vi "Read Attributes.vi"(11 "Set DER GenerationMode Msg":refnum<class "Set DER GenerationMode Msg.lvclass">) -> (2 "Payload":cluster{"DER_setGenerationMode":T1})   [LabVIEW 2018, in "Device Communication and Control Abstract Actor.lvlib" / "Set DER GenerationMode Msg.lvclass"]
uses:
  Set DER GenerationMode Msg.lvclass
  <vilib>/ORNL/CSEISMIC DDS/CSEISMIC DDS Base/Data Types/DER_setGenerationMode.ctl
  <vilib>/ORNL/CSEISMIC DDS/CSEISMIC DDS Base/Data Types/Controls/DeviceID.ctl
  <vilib>/ORNL/CSEISMIC DDS/CSEISMIC DDS Base/Data Types/Controls/Generation Mode.ctl
  Set DER GenerationMode Msg.lvclass/Set DER GenerationMode Msg.ctl
  <vilib>/ORNL/CSEISMIC DDS/CSEISMIC DDS Base/CSEISMIC DDS.lvclass
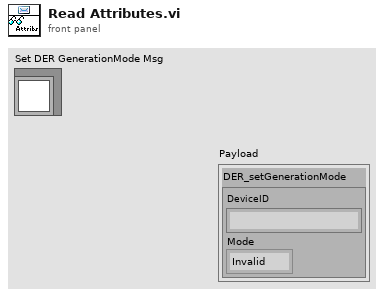
[diagram p1: front panel]
types:
  T1 = typedef "CSEISMIC DDS.lvlib/CSEISMIC DDS.lvclass/DER_setGenerationMode.ctl" = cluster{"DeviceID":T2, "Mode":T3}
  T2 = typedef "CSEISMIC DDS.lvlib/CSEISMIC DDS.lvclass/DeviceID.ctl" = string
  T3 = typedef "CSEISMIC DDS.lvlib/CSEISMIC DDS.lvclass/Generation Mode.ctl" = enum32{"Invalid", "PQ", "Droop", "PV", "PF", "VF"}
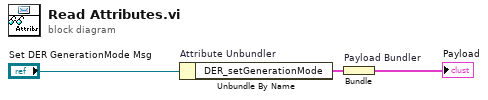
[diagram p0: block diagram]
diagram:
  n1 = Unbundle By Name "Attribute Unbundler"("Set DER GenerationMode Msg") -> ("DER_setGenerationMode"=w1:T1)
  n2 = Bundle "Payload Bundler"("DER_setGenerationMode"=w1) -> (→"Payload":cluster{"DER_setGenerationMode":T1})  [unwired: 1 in]
